vi "题目二.vi"() -> ()   [LabVIEW 2017]
panel:
  out "数值":i32
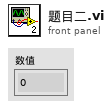
[diagram p1: front panel]
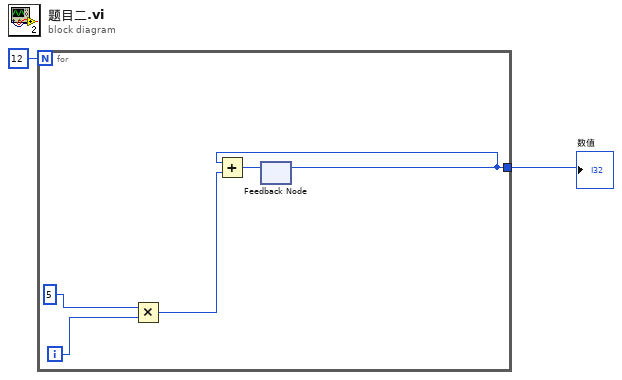
[diagram p0: block diagram]
diagram:
  n1 = for {
    N: 12 -> [_]
    tunnel: [w3] -> w1
    i -> [w6]
    n2 = Multiply(x=5, y=w6) -> (x*y=w5:i32)
    n3 = feedback #1() -> (w3:i32)  [unwired: 1 in]
    n4 = Add(x=w3, y=w5) -> (x+y=w4:i32)
    n5 = feedback-in #1(w4) -> ()
  }
  "数值" <- w1
